vi "Display Error.vi"(7 "type of dialog (OK msg:1)":T1=2 items=["no dialog", "OK message", "continue or stop message", "OK message + warnings", "continue/stop + warnings"], 8 "error in (no error)":errorcluster) -> (0 "error out":errorcluster, 3 "message":string=" INSTRUCTIONS:\r\rNormal Use:  When using subVIs that incorporate the error in/error out (or error I/O) structure, place this handler where you want to inform the user of an error, typically at the end of the I/O data path, as the last action of the program.  If the error in error? is ERROR, the handler creates a message describing the error and its source.  If the type of dialog = 1 (default), the message is displayed to the user, who can only acknowedge it.  If the type = 2, the user can acknowledge the message or abort execution; aborting a program with active I/O is not recommended.  If the type = 0, no message is displayed; this is used to process the error programmatically, and the error out cluster elements are wired to individual terminals for that reason.  \r\rOther Use:\n\r\nlocal testing.  To test the error code of a subVI or function that does not have the error I/O structure, you can wire its error code and a source string to the local error code and error source inputs.  If error in error? indicates no error and error code is not equal to 0, the local code and source are substituted for the error in values, and error? is set TRUE (ERROR).")   [LabVIEW 2018, in "Utilities.lvlib"]
uses:
  Utilities.lvlib
  <vilib>/Utility/error.llb/DialogType.ctl
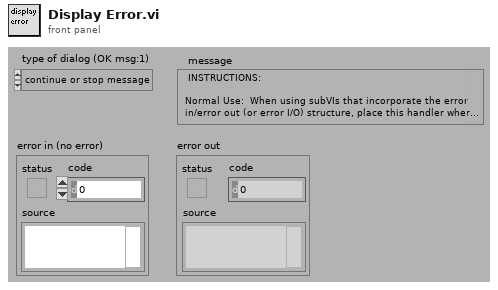
[diagram p1: front panel]
types:
  T1 = typedef "DialogType.ctl" = u16
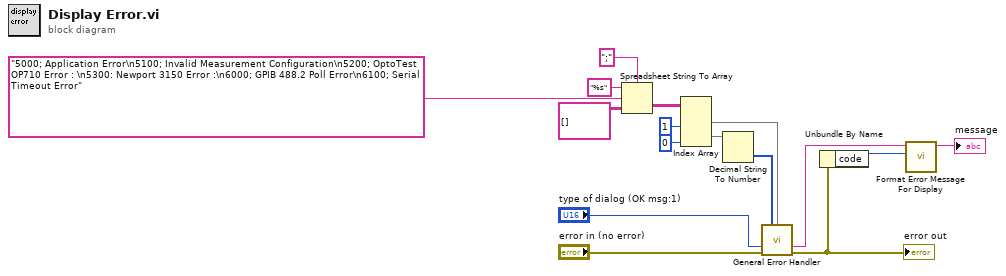
[diagram p0: block diagram]
diagram:
  n1 = Spreadsheet String To Array(delimiter (Tab)=";", format string="%s", spreadsheet string="5000; Application Error\n5100; Invalid Measurement Configuration\n5200; OptoTest OP710 Error : \n5300: Newport 3150 Error :\n6000; GPIB 488.2 Poll Error\n6100; Serial Timeout Error", array type (2D Dbl)=string[][] []) -> (array=w11:string[][])
  n2 = Index Array(array=w11, index (col) #1=1 ("disabled index (col)"), index (col) #2=0 ("index (col)")) -> (element #1=w5:string[], element #2=w7:string[])  [unwired: 2 in]
  n3 = Decimal String To Number(string=w7) -> (number=w6:i32[])  [unwired: 2 in, 1 out]
  n4 = call <vilib>:"General Error Handler.vi"("[user-defined codes]"=w6, "[user-defined descriptions]"=w5, "type of dialog (OK msg:1)"="type of dialog (OK msg:1)", "error in (no error)"="error in (no error)") -> ("message"=w4:string, "error out"=w3:errorcluster)  [unwired: 7 in, 3 out]
  "error out" <- w3
  n5 = Unbundle By Name(w3) -> ("code"=w2:i32)
  n6 = call "Format Error Message For Display.vi"("Error Code"=w2, "Error message"=w4) -> ("Display Message"=→"message":string)  [unwired: 9 in]
